vi "Show Triggers.vi"(8 "error in (no error)":errorcluster, 11 "Display State In":T1 caption="State") -> (0 "error out":errorcluster, 3 "Display State Out":T1 caption="State")   [LabVIEW 2020, in "PXISlotGP.xctl"]
uses:
  PXISlotGP.xctl
  State.ctl
  PXISlot XControl/Connector Type.ctl
  AOAIRefs.ctl
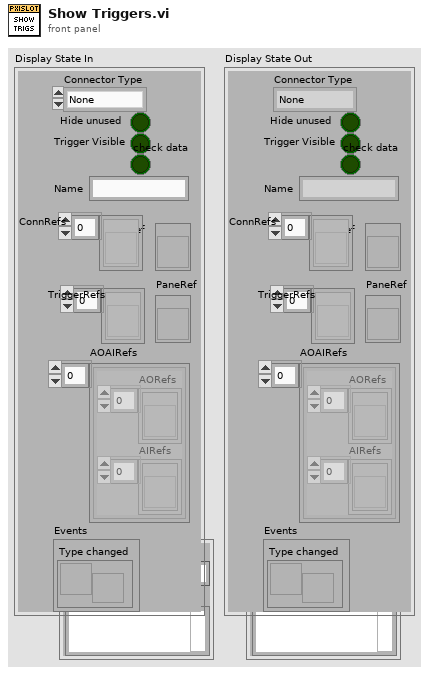
[diagram p1: front panel]
types:
  T1 = typedef "PXISlotGP.xctl/State.ctl" = cluster{"Connector Type":T2, "Hide unused":bool, "Trigger Visible":bool, "TabRef":refnum<vi>, "ConnRefs":refnum<vi>[], "PaneRef":refnum<vi>, "AOAIRefs":T3[], "TriggerRefs":refnum<vi>[], "check data":bool, "Name":string, "Events":cluster{"Type changed":refnum<user-event>}}
  T2 = typedef "Connector Type.ctl" = enum16{"None", "PXI-4461", "BNC-2110", "BNC-2090", "PXIe-4463", "PXIe-4464"}
  T3 = typedef "AOAIRefs.ctl" = cluster{"AORefs":refnum<vi>[], "AIRefs":refnum<vi>[]}
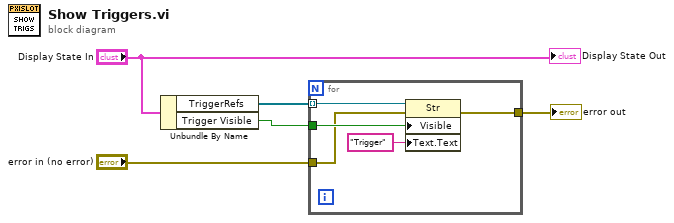
[diagram p0: block diagram]
diagram:
  n1 = Unbundle By Name("Display State In") -> ("TriggerRefs"=w3:refnum<vi>[], "Trigger Visible"=w4:bool)
  n2 = for {
    tunnel: w4 -> [w10]
    tunnel: w3 -> [w8] mode=indexing
    tunnel: "error in (no error)" -> [w7]
    tunnel: [w6] -> w1
    n3 = property class="Str"(reference=w8, error in=w7, "Visible"=w10, "Text.Text"="Trigger" ("Label.Text")) -> (error out=w6:errorcluster)  [unwired: 1 out]
  }
  "error out" <- w1
  "Display State Out" <- "Display State In"
